vi "read_attributes.vi"(8 "error in (no error)":errorcluster, 11 "MultiTaskElasticNet in":refnum<class "MultiTaskElasticNet.lvclass">) -> (0 "error out":errorcluster, 2 "attributes":T1, 3 "MultiTaskElasticNet out":refnum<class "MultiTaskElasticNet.lvclass">)   [LabVIEW 2020, in "MultiTaskElasticNet.lvclass"]
uses:
  MultiTaskElasticNet.lvclass
  Controls/multi_task_elastic_net_attributes.ctl
  MultiTaskElasticNet.lvclass/MultiTaskElasticNet.ctl
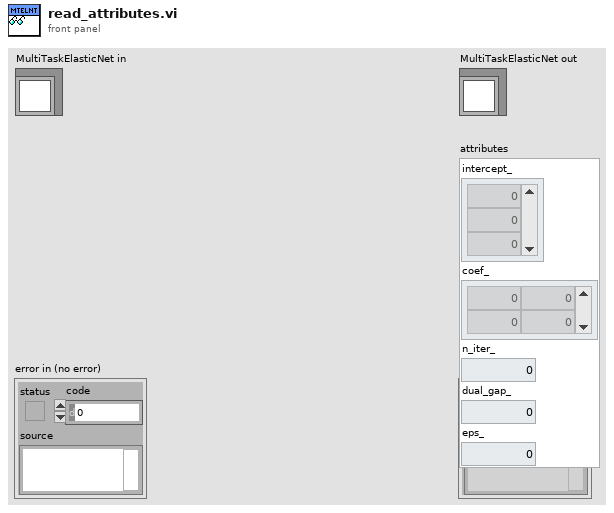
[diagram p1: front panel]
types:
  T1 = typedef "multi_task_elastic_net_attributes.ctl" = cluster{"intercept_":dbl[], "coef_":dbl[][], "n_iter_":dbl, "dual_gap_":dbl, "eps_":dbl}
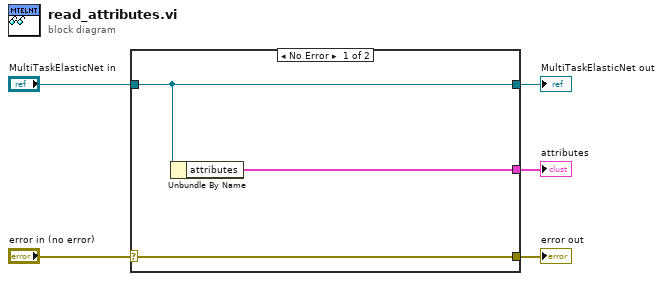
[diagram p0: block diagram]
diagram:
  n1 = case shown="No Error" "error in (no error)" {
    selector: "error in (no error)" -> [w8 w9]
    tunnel: [w8 w9] -> w4
    tunnel: [w7 w10] -> w2
    tunnel: "MultiTaskElasticNet in" -> [w7 w10]
    tunnel: [w6 _] -> w1
    frame No Error {
      n2 = Unbundle By Name(w7) -> ("attributes"=w6:T1)
    }
    frame Error {
    }
  }
  "error out" <- w4
  "MultiTaskElasticNet out" <- w2
  "attributes" <- w1
